vi "Launch.vi"(5 "window position":cluster{"Left":i16, "Top":i16}, 7 "options":T1, 8 "error in (no error)":errorcluster, 11 "Thread in":refnum<class "Thread.lvclass">) -> (0 "error out":errorcluster, 3 "Thread out":refnum<class "Thread.lvclass">)   [LabVIEW 2017, in "DSF Core.lvlib" / "Thread.lvclass"]
uses:
  Thread.lvclass
  DSF Thread Options.ctl
  Thread.lvclass/Thread.ctl
  DSF Core.lvlib
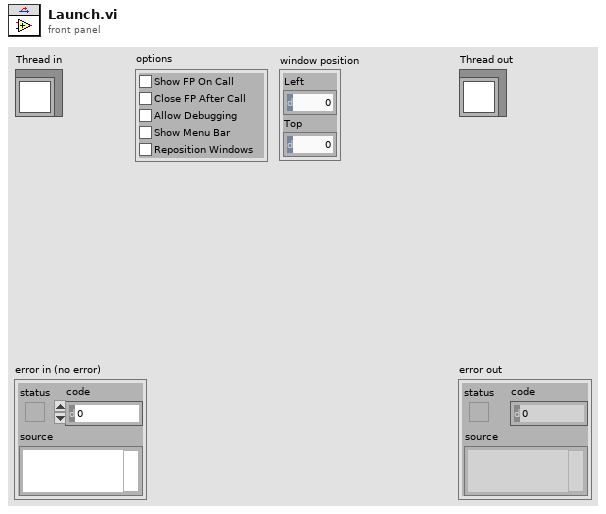
[diagram p1: front panel]
types:
  T1 = typedef "DSF Core.lvlib/DSF Thread Options.ctl" = cluster{"Show FP On Call":bool, "Close FP After Call":bool, "Allow Debugging":bool, "Show Menu Bar":bool, "Reposition Windows":bool}
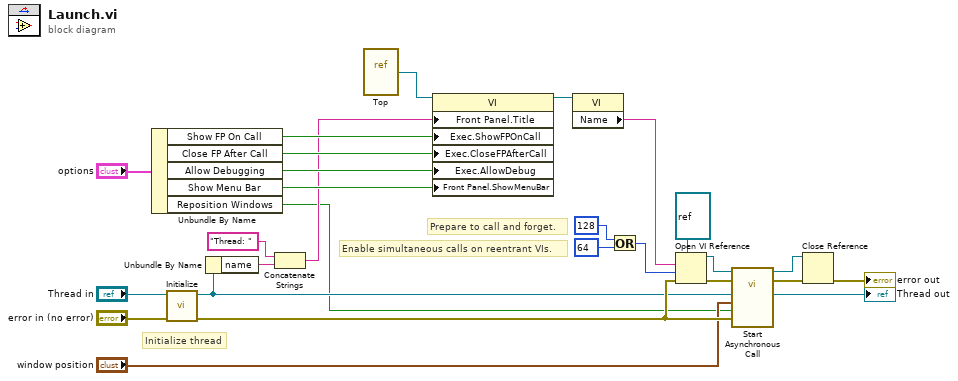
[diagram p0: block diagram]
diagram:
  # "Initialize thread"
  # "Prepare to call and forget."
  # "Enable simultaneous calls on reentrant VIs."
  n1 = Unbundle By Name("options") -> ("Show FP On Call"=w3:bool, "Close FP After Call"=w18:bool, "Allow Debugging"=w5:bool, "Show Menu Bar"=w4:bool, "Reposition Windows"=w1:bool)
  n2 = call-dynamic "Initialize.vi"("error in (no error)"="error in (no error)", "Thread in"="Thread in") -> ("error out"=w13:errorcluster, "Thread out"=w11:refnum<class "Thread.lvclass">)  [unwired: 8 in]
  "Thread out" <- w11
  n3 = Unbundle By Name(w11) -> ("name"=w14:string)
  n4 = Concatenate Strings("Thread: " ("string"), w14) -> (w2:string)
  n5 = vi-ref "Top.vi"() -> (w12:refnum<vi>)
  n6 = property class="VI"(reference=w12, "Front Panel.Title"=w2, "Exec.ShowFPOnCall"=w3, "Exec.CloseFPAfterCall"=w18, "Exec.AllowDebug"=w5, "Front Panel.ShowMenuBar"=w4) -> (reference out=w20:refnum<vi>)  [unwired: 1 in, 1 out]
  n7 = property class="VI"(reference=w20) -> ("Name"=w21:string)  [unwired: 1 in, 2 out]
  n8 = Or(x=128 ("options"), y=64 ("options")) -> (x .or. y?=w23:i32)
  n9 = Open VI Reference(type specifier VI Refnum (for type only)=refnum<vi> refnum, vi path=w21, options=w23, error in (no error)=w13) -> (vi reference=w9:refnum<vi>, error out=w10:errorcluster)  [unwired: 2 in]
  n10 = call-by-ref "Start Asynchronous Call"(reference=w9, error in=w10, 8:"error in (no error)"=w13, "reposition window"=w1, "window position"="window position", "Thread in"=w11) -> (reference out=w7:refnum<vi>, error out=w8:errorcluster)  [unwired: 6 in, 2 out]
  n11 = Close Reference(reference=w7, error in (no error)=w8) -> (error out=→"error out":errorcluster)
